vi "generate waiting time line.vi"(8 "每步等待时间(s)":dbl[](array[numeric]), 9 "阶段终点":dbl[](array[numeric]), 10 "FR zmag":dbl[](array[numeric]), 11 "真 终点":dbl) -> (2 "FR time line":dbl[](array[numeric]))   [LabVIEW 2017]
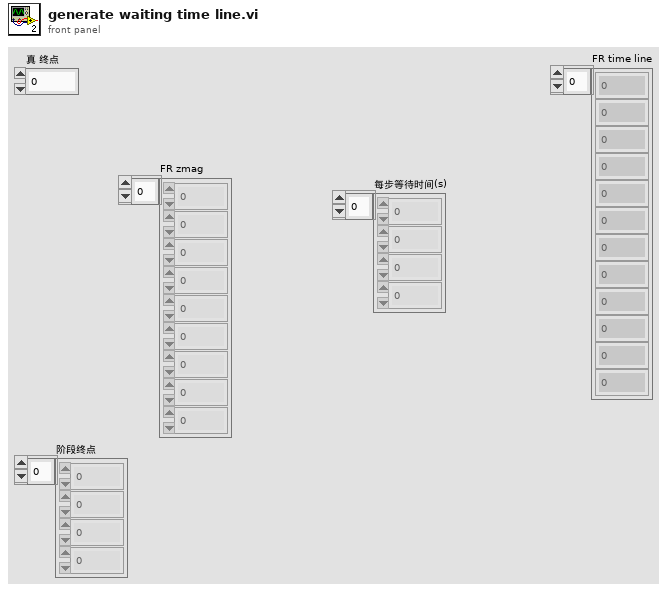
[diagram p1: front panel]
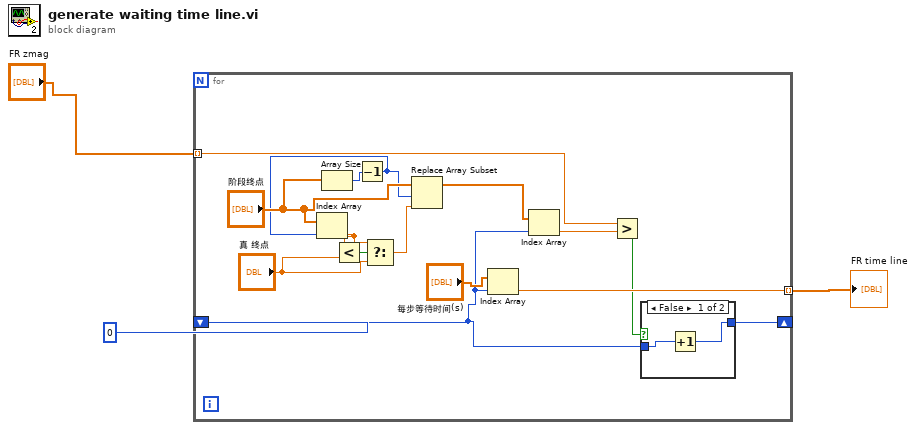
[diagram p0: block diagram]
diagram:
  n1 = for {
    tunnel: "FR zmag" -> [w16] mode=indexing
    shift-right: [w12] -> _
    shift-left: 0 -> [w13]
    tunnel: [w17] -> w1 mode=indexing
    n2 = Array Size(array="阶段终点") -> (size(s)=w11:i32)
    n3 = Decrement(x=w11) -> (x-1=w8:i32)
    n4 = Index Array(array="阶段终点", index=w8) -> (element=w6:dbl)
    n5 = Less?(x=w6, y="真 终点") -> (x < y?=w7:bool)
    n6 = Select(t=w6, s=w7, f="真 终点") -> (s? t:f=w4:dbl)
    n7 = Replace Array Subset(array="阶段终点", new element=w4, index=w8) -> (w10:dbl[])
    n8 = Index Array(array="每步等待时间(s)", index=w13) -> (element=w17:dbl)
    n9 = Index Array(array=w10, index=w13) -> (element=w15:dbl)
    n10 = Greater?(x=w16, y=w15) -> (0:w14:bool)
    n11 = case shown="False" w14 {
      tunnel: w13 -> [w20 w21]
      tunnel: [w19 w21] -> w12
      frame False {
        n12 = Increment(x=w20) -> (x+1=w19:i32)
      }
      frame True {
      }
    }
  }
  "FR time line" <- w1
